vi "MeasuringDevice.SetMeasurementBufferDepedency.vi"(8 "error in (no error)":errorcluster, 10 "CircularBuffer":refnum<class "CircularBuffer.lvclass">, 11 "MeasuringDevice":refnum<class "MeasuringDevice.lvclass">) -> (0 "error out":errorcluster, 3 "MeasuringDevice":refnum<class "MeasuringDevice.lvclass">)   [LabVIEW 2017, in "MeasuringDevice.lvclass"]
uses:
  MeasuringDevice.lvclass
  CircularBuffer/CircularBuffer.lvclass
  MeasuringDevice.lvclass/MeasuringDevice.ctl
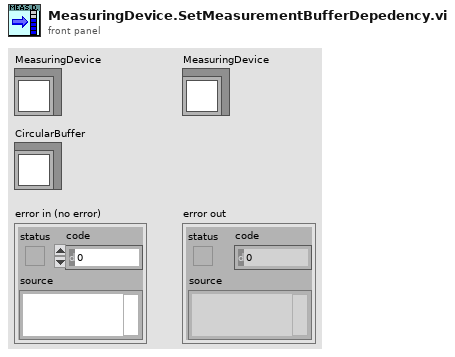
[diagram p1: front panel]
types:
  T1 = typedef "MeasuringDevice.lvclass/PrivateData--Ref.ctl" = refnum<data-value>
  T2 = typedef "MeasuringDevice.lvclass/PrivateData--Cluster.ctl" = cluster{"Public Events":T3, "Private Events":T4, "Dependencies":T5}
  T3 = typedef "MeasuringDevice.lvclass/PublicEvents--Cluster.ctl" = cluster{"MeasurementCompleted":refnum<user-event>}
  T4 = typedef "MeasuringDevice.lvclass/PrivateEvents--Cluster.ctl" = cluster{"MakeMeasurement":refnum<user-event>}
  T5 = typedef "MeasuringDevice.lvclass/Dependencies--Cluster.ctl" = cluster{"MeasurementBuffer":refnum<class "CircularBuffer.lvclass">}
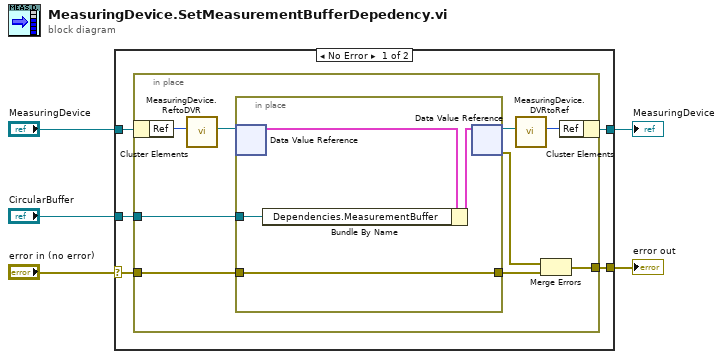
[diagram p0: block diagram]
diagram:
  n1 = case shown="No Error" "error in (no error)" {
    selector: "error in (no error)" -> [w7 w24]
    tunnel: "MeasuringDevice" -> [w10 w25]
    tunnel: [w9 w25] -> w3
    tunnel: "CircularBuffer" -> [w8 _]
    tunnel: [w6 w24] -> w1
    frame No Error {
      n2 = in-place {
        in-place-border: w8 -> [w15]
        in-place-border: w7 -> [w14]
        in-place-border: [w11] -> w6
        n3 = in-place-cluster #1(w10) -> ("Ref"=w19:u32)
        n4 = call "MeasuringDevice.ReftoDVR.vi"("Ref"=w19) -> ("Ref"=w17:T1)  [unwired: 10 in]
        n5 = in-place {
          in-place-border: w15 -> [w22]
          in-place-border: w14 -> [w20]
          in-place-border: [w20] -> w13
          n6 = in-place-dvr #2(w17) -> (w23:T2)  [unwired: 1 out]
          n7 = Bundle By Name(cluster=w23, "Dependencies.MeasurementBuffer"=w22) -> (w21:T2)
          n8 = in-place-dvr #2(w21) -> (w16:T1, w12:errorcluster)
        }
        n9 = call "MeasuringDevice.DVRtoRef.vi"("Ref"=w16) -> ("Ref"=w18:u32)  [unwired: 10 in]
        n10 = Merge Errors(w12, w13) -> (w11:errorcluster)
        n11 = in-place-cluster #1("Ref"=w18) -> (w9:refnum<class "MeasuringDevice.lvclass">)
      }
    }
    frame Error {
    }
  }
  "error out" <- w1
  "MeasuringDevice" <- w3
